vi "magnet position sweep and PL read.vi"() -> ()   [LabVIEW 2012]
uses:
  <vilib>/Analysis/1siggen.llb/Ramp Pattern by Samples.vi
  VELMEX step motor/GMW Motion Control_VELMEX_V2_2.llb/Config.vi
  <vilib>/Utility/file.llb/Write To Spreadsheet File (DBL).vi
  <vilib>/Analysis/NI_AALBase.lvlib
panel:
  in  "Time Target (s)":dbl=10.0
  in  "Z-track?":bool
  in  "Z Position 2":dbl
  in  "Y Position 2":dbl
  in  "X Position 2":dbl
  out "Average intensity (cts/s)":dbl
  in  "theta":dbl
  in  "Boolean":bool
  in  "file path (dialog if empty)":path
  out "transposed array":dbl[][](array[numeric])
  out "Z Position":sgl=6.0 format="%.2f"
  out "Y Position":sgl format="%.2f"
  out "X Position":sgl format="%.2f"
  out "Angle(T) Position":sgl=1.0 format="%.1f"
  in  "start":dbl format="%0.2f"
  in  "end":dbl=1.0 format="%0.2f"
  in  "samples":i32=128
  in  "GPIB Address":refnum<visa-resource-name>="GPIB0::1::INSTR"
  in  "datalog path (use dialog)":path
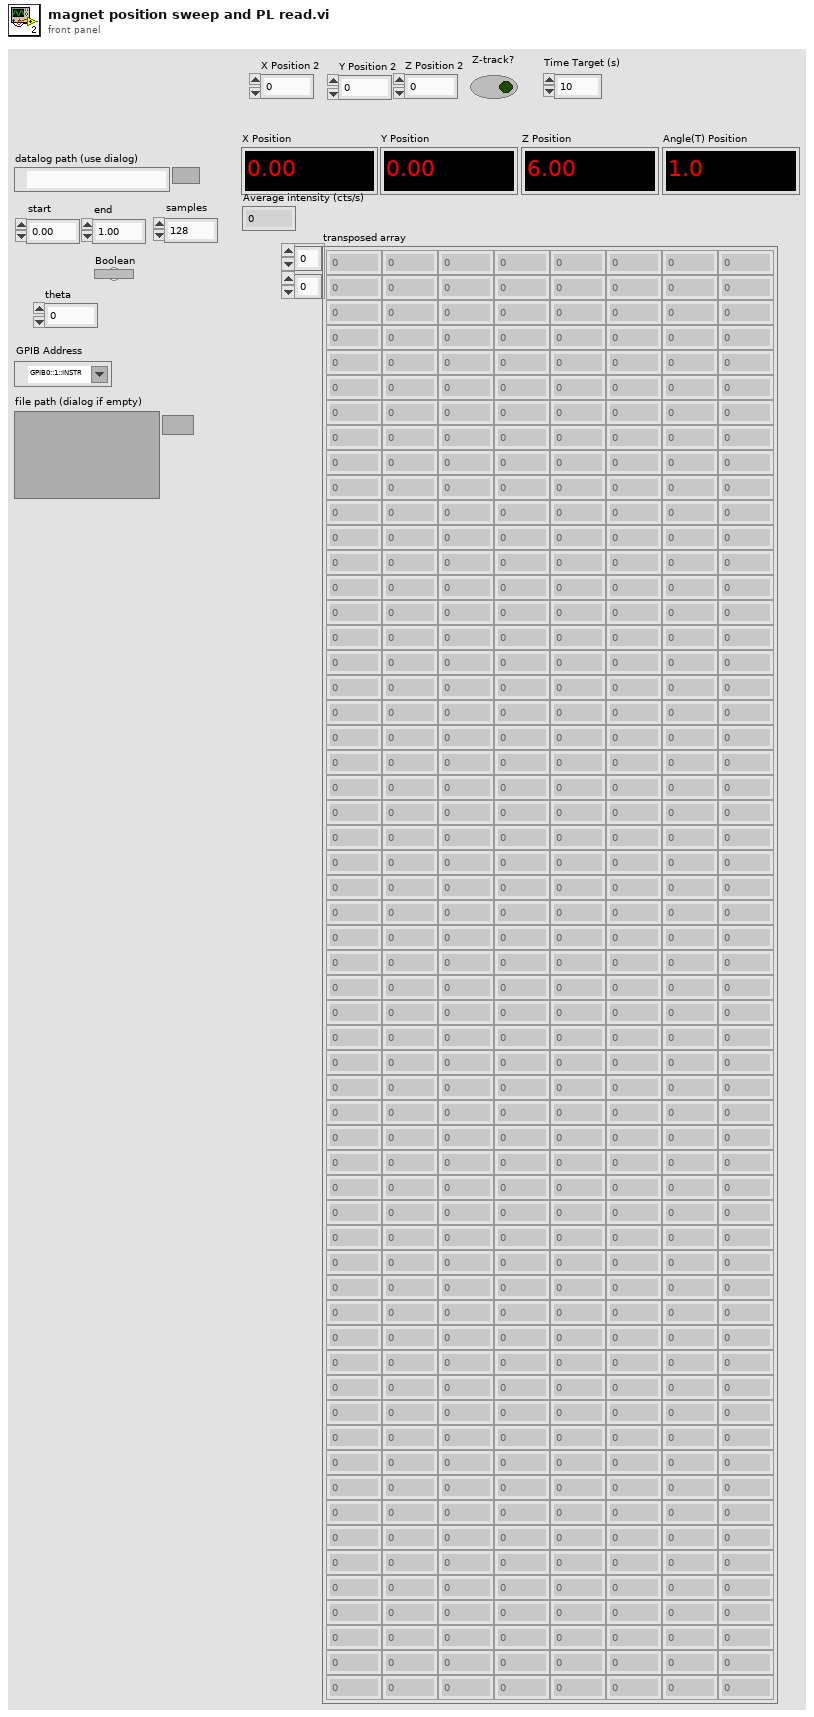
[diagram p1: front panel]
types:
  T1 = cluster{"Controller Setup":cluster{"T":string, "Z":string, "Y":string, "X":string, "CW Offset":dbl, "CCW Offset":dbl, "Z Offset":dbl, "Y Offset":dbl, "X Offset":dbl, "Rotary Resolution":i32, "Linear Resolution":i32, "T Speed":dbl, "Z Speed":dbl, "Y Speed":dbl, "X Speed":dbl}, "SoftLimit":cluster{"X soft limit":cluster{"X up soft limit":dbl, "X low soft limit":dbl}, "Y soft limit":cluster{"Y up soft limit":dbl, "Y low soft limit":dbl}, "Z soft limit":cluster{"Z up soft limit":dbl, "Z low soft limit":dbl}, "T soft limit":cluster{"T up soft limit":dbl, "T low soft limit":dbl}}}
  T2 = cluster{"T":string, "Z":string, "Y":string, "X":string, "CW Offset":dbl, "CCW Offset":dbl, "Z Offset":dbl, "Y Offset":dbl, "X Offset":dbl, "Rotary Resolution":i32, "Linear Resolution":i32, "T Speed":dbl, "Z Speed":dbl, "Y Speed":dbl, "X Speed":dbl}
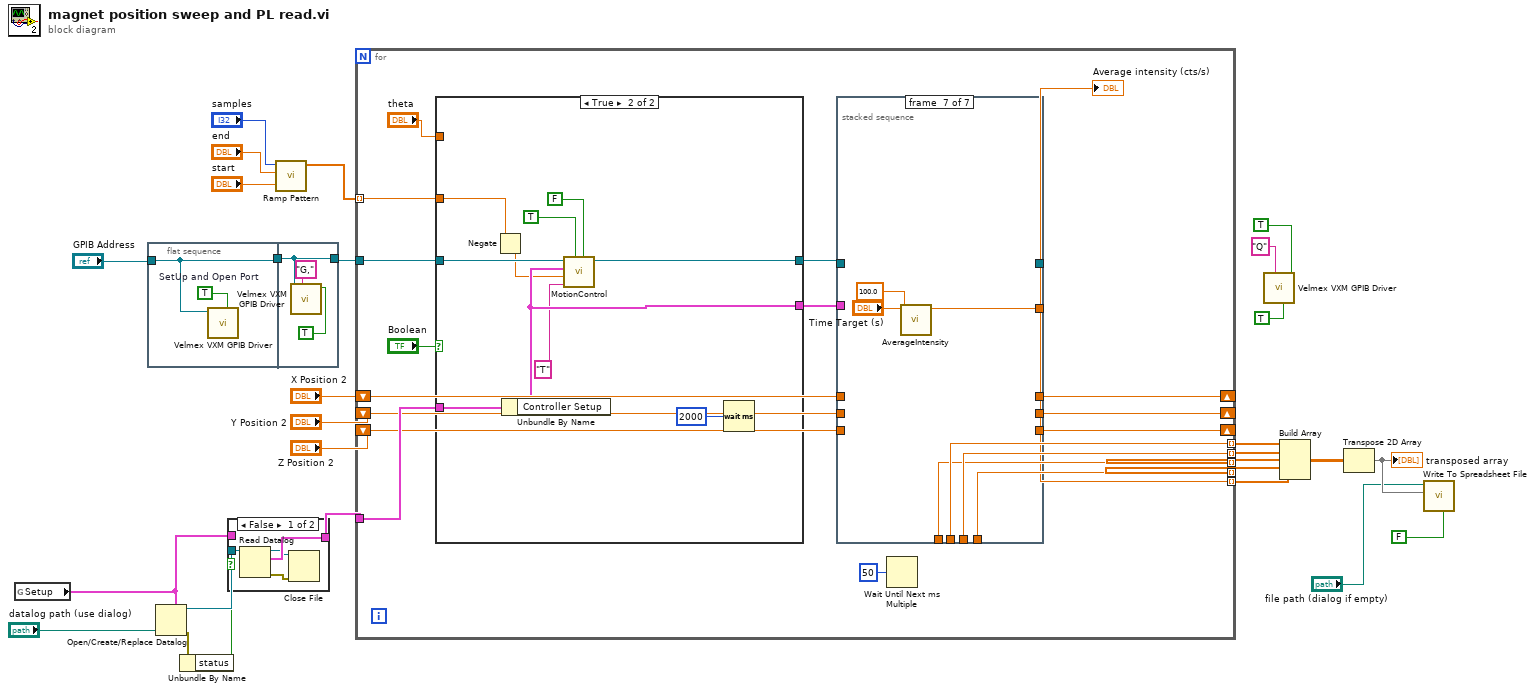
[diagram p0: block diagram]
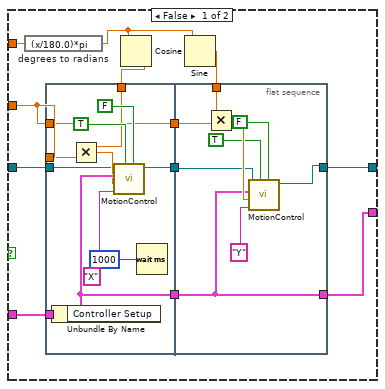
[diagram p2: hidden frame]
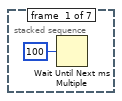
[diagram p3: hidden frame]
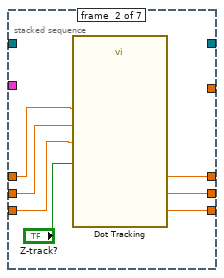
[diagram p4: hidden frame]
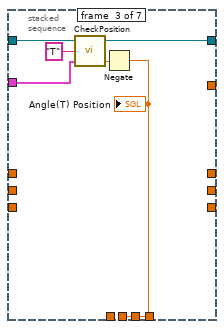
[diagram p5: hidden frame]
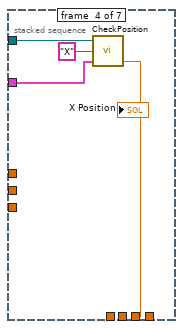
[diagram p6: hidden frame]
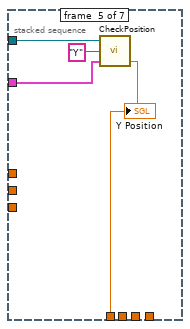
[diagram p7: hidden frame]
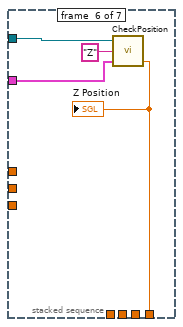
[diagram p8: hidden frame]
diagram:
  n1 = global read "Config.vi" "Setup"() -> (w26:T1)
  n2 = flat-sequence {
    tunnel: "GPIB Address" -> [w29]
    tunnel: [w29] -> w23
    tunnel: [w33] -> w18
    tunnel: w23 -> [w33]
    frame #0 {
      w30 = TRUE  # SetUp and Open Port
      n3 = call "Velmex VXM GPIB Driver.vi"("SetUp and Open Port"=w30, "VISA resource name"=w29) -> ()  [unwired: 8 in, 2 out]
    }
    frame #1 {
      n4 = call "Velmex VXM GPIB Driver.vi"("Send String to VXM"=TRUE, "String to send to VXM"="G,", "VISA resource name"=w33) -> ()  [unwired: 7 in, 2 out]
    }
  }
  n5 = Open/Create/Replace Datalog(5:w26, 11:"datalog path (use dialog)") -> (0:w28:errorcluster, 3:w27:refnum<k1>)  [unwired: 4 in, 1 out]
  n6 = Unbundle By Name(w28) -> ("status"=w25:bool)
  n7 = case shown="False" w25 {
    tunnel: w27 -> [w34 _]
    tunnel: [w37 w38] -> w17
    tunnel: w26 -> [_ w38]
    frame False {
      n8 = Read Datalog(7:w34) -> (0:w36:errorcluster, 2:w37:T1, 3:w35:refnum<k1>)  [unwired: 2 in]
      n9 = Close File(refnum=w35, error in=w36) -> ()  [unwired: 2 out]
    }
    frame True {
    }
  }
  n10 = call-poly <vilib>:"Ramp Pattern.vi"("start"="start", "end"="end", "samples"="samples") -> ("Ramp Pattern"=w13:dbl[])  [unwired: 7 in, 1 out]
  n11 = for {
    tunnel: w13 -> [w55] mode=indexing
    tunnel: w18 -> [w57]
    tunnel: w17 -> [w56]
    tunnel: [w52] -> w12 mode=indexing
    tunnel: [w51] -> w11 mode=indexing
    tunnel: [w50] -> w10 mode=indexing
    tunnel: [w49] -> w9 mode=indexing
    tunnel: [w47] -> w4 mode=indexing
    shift-right: [w44] -> _
    shift-left: "X Position 2" -> [w41]
    shift-right: [w43] -> _
    shift-left: "Y Position 2" -> [w40]
    shift-right: [w42] -> _
    shift-left: "Z Position 2" -> [w39]
    n12 = case shown="True" "Boolean" {
      tunnel: w57 -> [w68 w99]
      tunnel: w56 -> [w69 w98]
      tunnel: w55 -> [w59 w97]
      tunnel: [w61 w94] -> w54
      tunnel: [w62 w93] -> w53
      tunnel: "theta" -> [w65 _]
      frame False {
        n13 = expression code="(x/180.0)*pi" "degrees to radians"(w65) -> (w66:dbl)
        n14 = flat-sequence {
          tunnel: w69 -> [w77]
          tunnel: w68 -> [w70]
          tunnel: w67 -> [w75]
          tunnel: w59 -> [w73]
          tunnel: [w70] -> w64
          tunnel: [w76] -> w63
          tunnel: [w72] -> w60
          tunnel: w59 -> [w72]
          tunnel: [w85] -> w62
          tunnel: [w81] -> w61
          tunnel: w64 -> [w82]
          tunnel: w63 -> [w85]
          tunnel: w60 -> [w84]
          tunnel: w58 -> [w83]
          frame #0 {
            n15 = Unbundle By Name(w77) -> ("Controller Setup"=w76:T2)
            n16 = Multiply(x=w75, y=w73) -> (x*y=w74:dbl)
            n17 = call "MotionControl.vi"("STOP motion"=FALSE, "START motion"=TRUE, "axis"="X", "Position"=w74, "Setup"=w76, "VISA resource name in"=w70) -> ()  [unwired: 3 in, 1 out]
            n18 = Wait (ms)(milliseconds to wait=u32 1000) -> ()  [unwired: 1 out]
          }
          frame #1 {
            n19 = Multiply(x=w83, y=w84) -> (x*y=w89:dbl)
            n20 = call "MotionControl.vi"("STOP motion"=FALSE, "START motion"=TRUE, "axis"="Y", "Position"=w89, "Setup"=w85, "VISA resource name in"=w82) -> ("VISA resource name out"=w81:refnum<visa-resource-name>)  [unwired: 3 in]
          }
        }
        n21 = Cosine(x=w66) -> (cos(x)=w67:dbl)
        n22 = Sine(x=w66) -> (sin(x)=w58:dbl)
      }
      frame True {
        n23 = Negate(x=w97) -> (-x=w91:dbl)
        n24 = Unbundle By Name(w98) -> ("Controller Setup"=w93:T2)
        n25 = call "MotionControl.vi"("STOP motion"=FALSE, "START motion"=TRUE, "axis"="T", "Position"=w91, "Setup"=w93, "VISA resource name in"=w99) -> ("VISA resource name out"=w94:refnum<visa-resource-name>)  [unwired: 3 in]
        n26 = Wait (ms)(milliseconds to wait=u32 2000) -> ()  [unwired: 1 out]
      }
    }
    n27 = stacked-sequence {
      tunnel: [_ _ w108 _ _ _ _] -> _
      tunnel: w54 -> [_ _ w112 w116 w120 w124 _]
      tunnel: w53 -> [_ _ w111 w115 w119 w123 _]
      tunnel: [_ _ w109 _ _ _ _] -> w52
      tunnel: [_ _ _ w114 _ _ _] -> w51
      tunnel: [_ _ _ _ w118 _ _] -> w50
      tunnel: [_ _ _ _ _ w122 _] -> w49
      tunnel: [_ _ _ _ _ _ w127] -> w47
      tunnel: [_ w107 _ _ _ _ _] -> w44
      tunnel: [_ w106 _ _ _ _ _] -> w43
      tunnel: [_ w105 _ _ _ _ _] -> w42
      tunnel: w41 -> [_ w104 _ _ _ _ _]
      tunnel: w40 -> [_ w103 _ _ _ _ _]
      tunnel: w39 -> [_ w102 _ _ _ _ _]
      frame #0 {
        n28 = Wait Until Next ms Multiple(millisecond multiple=u32 100) -> ()  [unwired: 1 out]
      }
      frame #1 {
        n29 = call "Dot Tracking.vi"("X Pos"=w104, "Y pos"=w103, "Z Pos"=w102, "Z-track?"="Z-track?") -> ("X Position"=w107:dbl, "Y Position"=w106:dbl, "Z Position"=w105:dbl)  [unwired: 5 in, 4 out]
      }
      frame #2 {
        n30 = call "CheckPosition.vi"("Setup"=w111, "Input string"="T", "VISA resource name in"=w112) -> ("Position"=w110:sgl, "VISA resource name out"=w108:refnum<visa-resource-name>)  [unwired: 1 in]
        n31 = Negate(x=w110) -> (-x=w109:sgl)
        "Angle(T) Position" <- w109
      }
      frame #3 {
        n32 = call "CheckPosition.vi"("Setup"=w115, "Input string"="X", "VISA resource name in"=w116) -> ("Position"=w114:sgl)  [unwired: 1 in, 1 out]
        "X Position" <- w114
      }
      frame #4 {
        n33 = call "CheckPosition.vi"("Setup"=w119, "Input string"="Y", "VISA resource name in"=w120) -> ("Position"=w118:sgl)  [unwired: 1 in, 1 out]
        "Y Position" <- w118
      }
      frame #5 {
        n34 = call "CheckPosition.vi"("Setup"=w123, "Input string"="Z", "VISA resource name in"=w124) -> ("Position"=w122:sgl)  [unwired: 1 in, 1 out]
        "Z Position" <- w122
      }
      frame #6 {
        n35 = call "AverageIntensity.vi"("rate (Hz)"=100.0, "Time Target (s)"="Time Target (s)") -> ("Average intensity (cts/s)"=w127:dbl)  [unwired: 8 in, 1 out]
      }
    }
    "Average intensity (cts/s)" <- w47
    n36 = Wait Until Next ms Multiple(millisecond multiple=u32 50) -> ()  [unwired: 1 out]
  }
  n37 = call "Velmex VXM GPIB Driver.vi"("Send String to VXM"=TRUE, "Close Port"=TRUE, "String to send to VXM"="Q") -> ()  [unwired: 7 in, 2 out]
  n38 = Build Array(w12, w11, w10, w9, w4) -> (w8:dbl[][])
  n39 = Transpose 2D Array(2D array=w8) -> (transposed array=w7:dbl[][])
  "transposed array" <- w7
  n40 = call-poly <vilib>:"Write To Spreadsheet File.vi"("transpose? (no:F)"=FALSE, "2D data"=w7, "file path (dialog if empty)"="file path (dialog if empty)") -> ()  [unwired: 5 in, 1 out]
